vi "Labview_FFT_Orig.vi"(0 "Channel A":u16[][](array[numeric]), 5 "Range":dbl format="%#_13g", 7 "Bits":dbl) -> (4 "Int B-Scan Channel A":sgl[][](array[numeric]))   [LabVIEW 2016]
uses:
  <vilib>/Analysis/4window.llb/Hanning Window (DBL).vi
  <vilib>/Analysis/2dsp.llb/Real FFT.vi
  <vilib>/Analysis/4window.llb/AllCosWindow (DBL).vi
  <vilib>/Analysis/NI_AALPro.lvlib
panel:
  in  "Log10?":bool
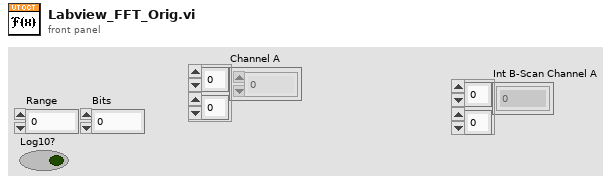
[diagram p1: front panel]
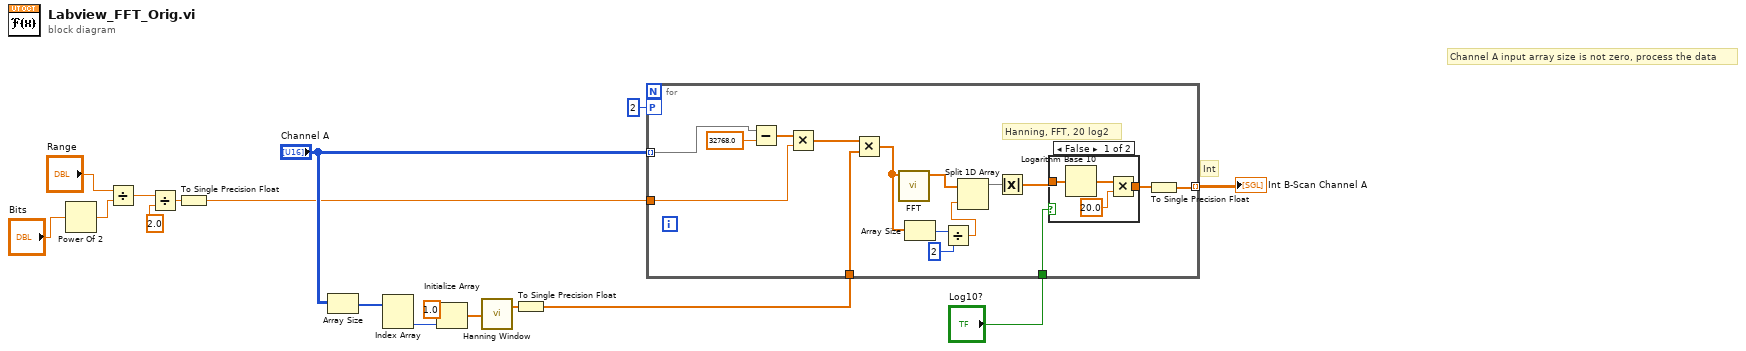
[diagram p0: block diagram]
diagram:
  # "Channel A input array size is not zero, process the data"
  # "Int"
  n1 = Power Of 2(x="Bits") -> (2^x=w17:dbl)
  n2 = Divide(x="Range", y=w17) -> (x/y=w16:dbl)
  n3 = Divide(x=w16, y=2.0) -> (x/y=w5:dbl)
  n4 = To Single Precision Float(number=w5) -> (single precision float=w3:sgl)
  n5 = Array Size(array="Channel A") -> (size(s)=w8:i32[])
  n6 = Index Array(array=w8) -> (element #2=w7:i32)  [unwired: 2 in, 1 out]
  n7 = Initialize Array(1.0 ("element"), w7) -> (w14:dbl[])
  n8 = call-poly <vilib>:"Hanning Window.vi"("X"=w14) -> ("Windowed X"=w4:dbl[])  [unwired: 1 out]
  n9 = To Single Precision Float(number=w4) -> (single precision float=w2:sgl[])
  n10 = for {
    tunnel: [w22] -> w1 mode=indexing
    tunnel: w2 -> [w25]
    workers-P: 2 -> [_]
    tunnel: w3 -> [w24]
    tunnel: "Channel A" -> [w23] mode=indexing
    tunnel: "Log10?" -> [w20]
    # "Hanning, FFT, 20 log2"
    n11 = Subtract(x=w23, y=32768.0 ("element")) -> (x-y=w27:dbl[])
    n12 = Multiply(x=w27, y=w24) -> (x*y=w26:dbl[])
    n13 = Multiply(x=w26, y=w25) -> (x*y=w29:dbl[])
    n14 = call-poly <vilib>:"FFT.vi"("X"=w29) -> ("FFT {X}"=w30:cdb[])  [unwired: 9 in, 1 out]
    n15 = Array Size(array=w29) -> (size(s)=w33:i32)
    n16 = Divide(x=w33, y=2) -> (x/y=w31:dbl)
    n17 = Split 1D Array(array=w30, index=w31) -> (first subarray=w18:cdb[])  [unwired: 1 out]
    n18 = Absolute Value(x=w18) -> (abs(x)=w19:dbl[])
    n19 = case shown="False" w20 {
      tunnel: w19 -> [w37 w38]
      tunnel: [w34 w38] -> w21
      frame False {
        n20 = Logarithm Base 10(1:w37) -> (0:w36:dbl[])
        n21 = Multiply(x=w36, y=sgl 20.0) -> (x*y=w34:dbl[])
      }
      frame True {
      }
    }
    n22 = To Single Precision Float(number=w21) -> (single precision float=w22:sgl[])
  }
  "Int B-Scan Channel A" <- w1
